vi "readfromsv.vi"() -> (3 "Cluster":T1 {"mode" items=["classic", "countdown", "ai"]; "player"."status" items=["host_ready", "idle", "host", "leaved", "ready", "playing", "lose(mine)", "lose(ot)", "win"]})   [LabVIEW 2025]
uses:
  gbv.vi
  controls/playerstatus.ctl
  multi.ctl
panel:
  out "error out":errorcluster
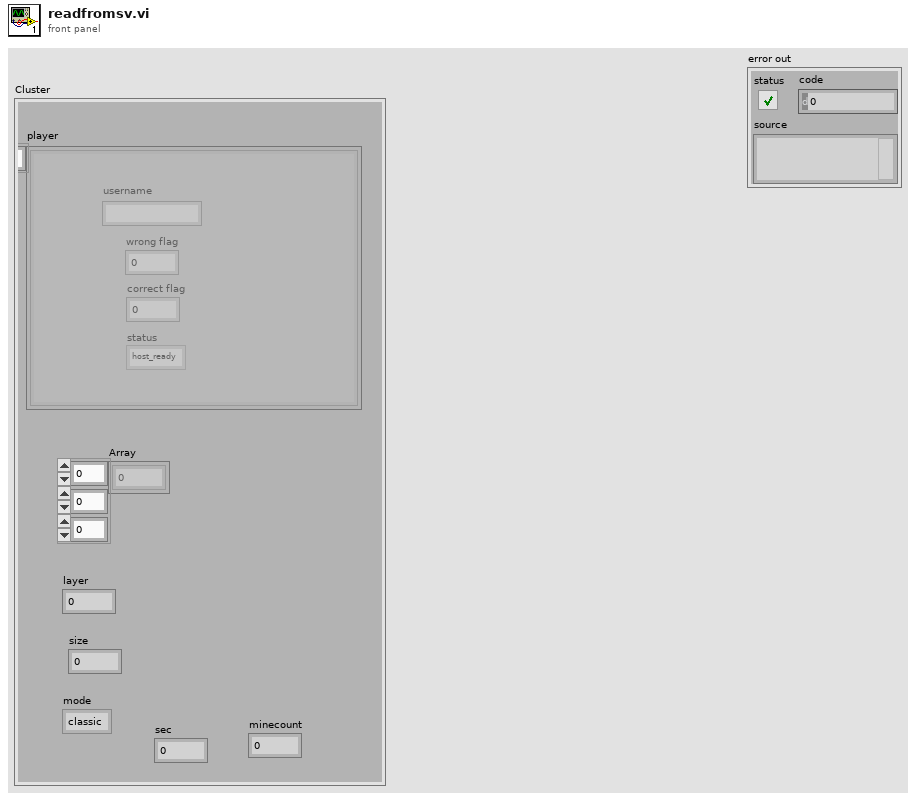
[diagram p1: front panel]
types:
  T1 = typedef "multi.ctl" = cluster{"Array":i8[][][], "player":T2[], "layer":i32, "size":i32, "mode":u16, "sec":i32, "minecount":i32}
  T2 = typedef "playerstatus.ctl" = cluster{"correct flag":i32, "wrong flag":i32, "username":string, "status":u16}
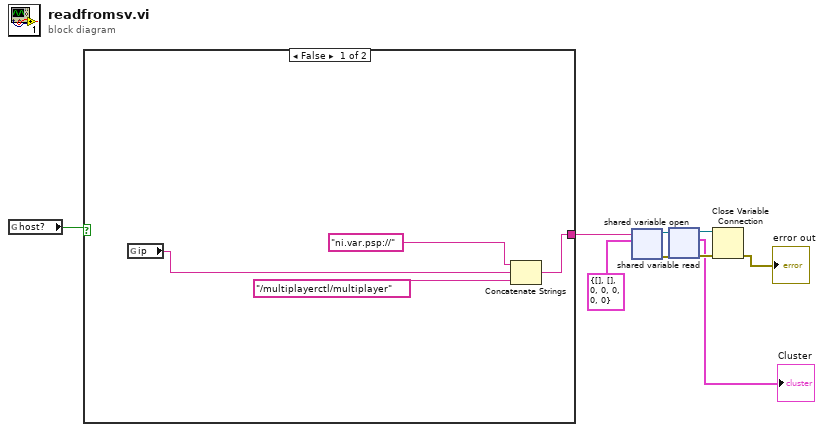
[diagram p0: block diagram]
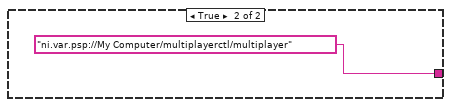
[diagram p2: hidden frame]
diagram:
  n1 = global read "gbv.vi" "host?"() -> (w9:bool)
  n2 = case shown="False" w9 {
    tunnel: [w10 "ni.var.psp://My Computer/multiplayerctl/multiplayer"] -> w8
    frame False {
      n3 = global read "gbv.vi" "ip"() -> (w11:string)
      n4 = Concatenate Strings("ni.var.psp://" ("string"), w11, "/multiplayerctl/multiplayer" ("string")) -> (w10:string)
    }
    frame True {
    }
  }
  n5 = shared-variable-open(w8, T1 {"Array"=[], "player"=[], "layer"=0, "size"=0, "mode"=0, "sec"=0, "minecount"=0} ("multiplayer")) -> (w6:refnum<k21>, w5:errorcluster)  [unwired: 2 in]
  n6 = shared-variable-read(w6, w5) -> (w3:refnum<k21>, w4:errorcluster, →"Cluster":T1)  [unwired: 1 out]
  n7 = Close Variable Connection(8:w4, 11:w3) -> (0:→"error out":errorcluster)
